vi "Perform Checks.vi"(4 "Owner Path (if applicable)":path, 6 "User VI Owner Status":T1, 8 "error in":errorcluster, 10 "Selected Template VI or CTL name (including file extension)":string, 11 "Destination Folder":path) -> (0 "error out":errorcluster)   [LabVIEW 2021]
doc: "Performs a few sanity checks in order to ensure that everything is ok before attempting to create a new VI based on these inputs. In other words, performs input validation.\n\nSanity checks:\n1. Destination folder exists\n2. Destination folder does not already contain a file with the same name and extension as is about to be created\n3. Selected Template VI or CTL exists\n4. Owner Library or Class exists (if applicable, meaning if the User VI was owned by a library or class)\n\nReturns a meaningful, informative error if any of the sanity checks failed."
uses:
  Owner Status (enum).ctl
panel:
  # "Development\ncontrols/indicators useful for development and testing, but which are not outputs of the VI"
  # "Input\nInputs to the VI"
  # "Output\nOutputs of the VI"
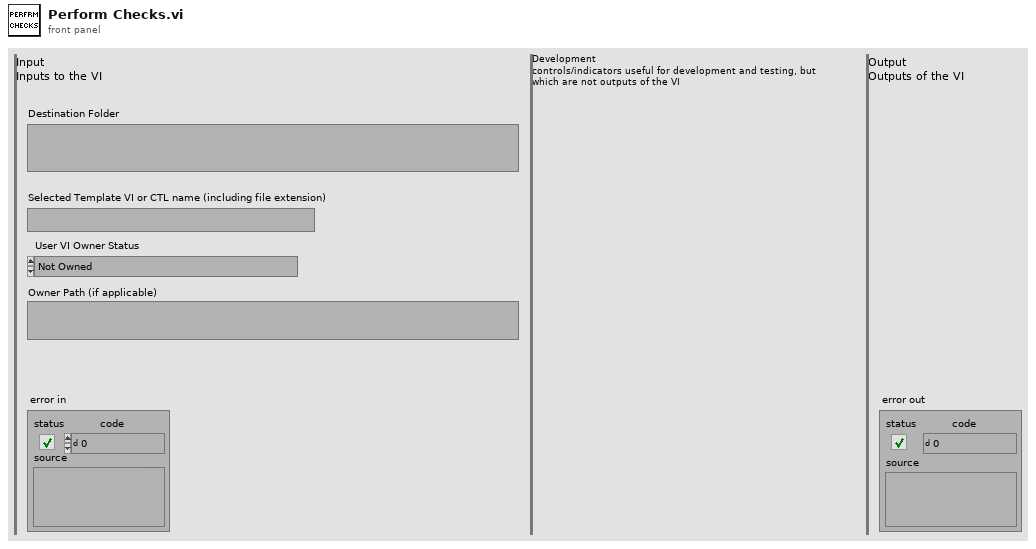
[diagram p1: front panel]
types:
  T1 = typedef "Owner Status (enum).ctl" = enum16{"Not Owned", "Owned by Library (lvlib)", "Owned by Class (lvclass)"}
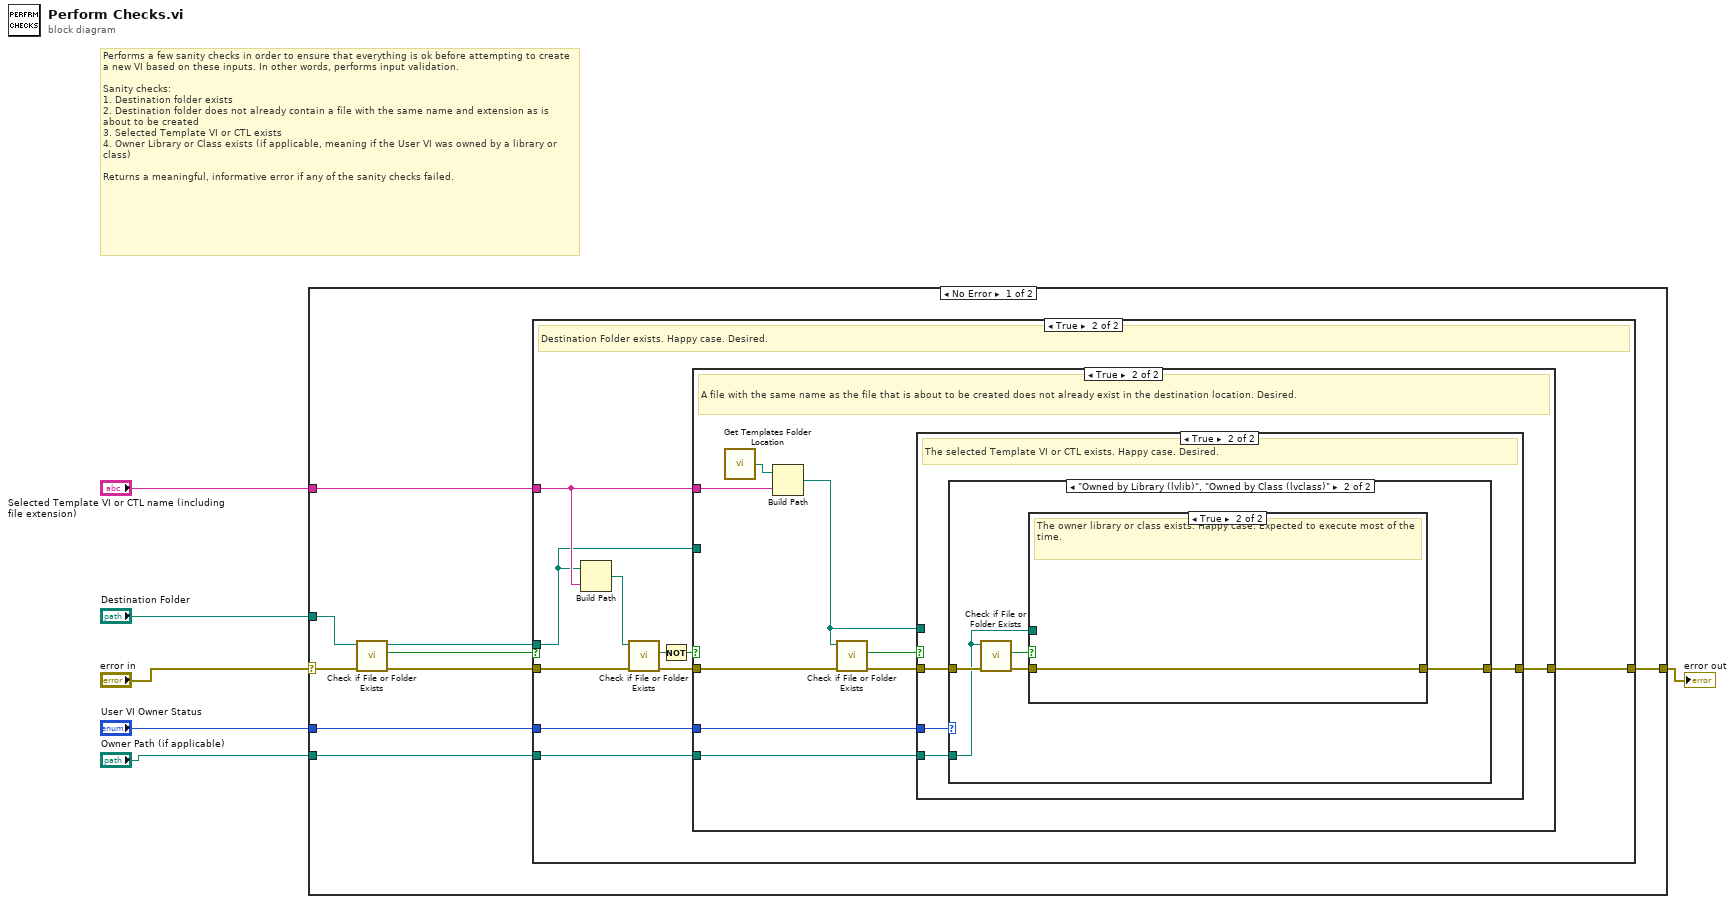
[diagram p0: block diagram]
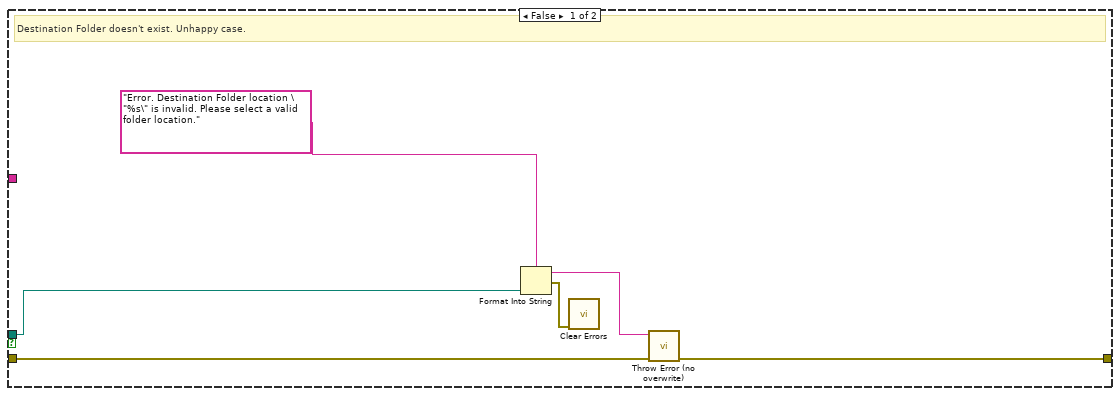
[diagram p2: hidden frame]
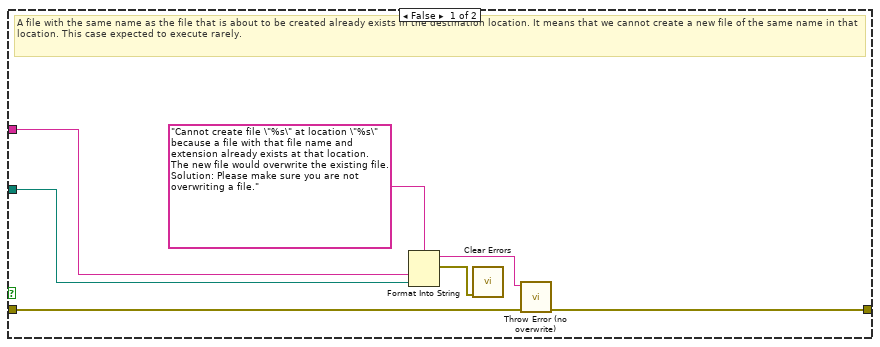
[diagram p3: hidden frame]
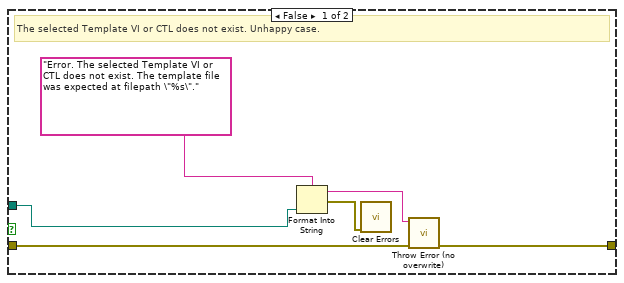
[diagram p4: hidden frame]
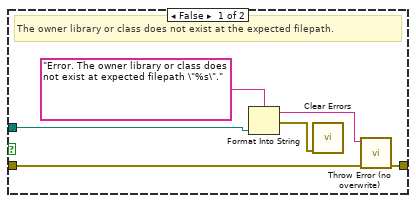
[diagram p6: hidden frame]
diagram:
  # "Performs a few sanity checks in order to ensure that everything is ok before attempting to create a new VI based on these inputs. In other words, performs input validation.\n\nSanity checks:\n1. Destination folder exists\n2. Destination folder does not already contain a file with the same name and extension as is about to be created\n3. Selected Template VI or CTL exists\n4. Owner Library or Class exists (if applicable, meaning if the User VI was owned by a library or class)\n\nReturns a meaningful, informative error if any of the sanity checks failed."
  n1 = case shown="No Error" "error in" {
    selector: "error in" -> [w14 w71]
    tunnel: [w11 w71] -> w5
    tunnel: "Destination Folder" -> [w15 _]
    tunnel: "Selected Template VI or CTL name (including file extension)" -> [w9 _]
    tunnel: "User VI Owner Status" -> [w8 _]
    tunnel: "Owner Path (if applicable)" -> [w7 _]
    frame No Error {
      n2 = call <vilib>:"Check if File or Folder Exists.vi"("error in (no error)"=w14, "path"=w15) -> ("error out"=w13:errorcluster, "file or folder exists?"=w12:bool, "dup path"=w10:path)  [unwired: 7 in]
      n3 = case shown="True" w12 {
        tunnel: w13 -> [w21 w26]
        tunnel: [w20 w31] -> w11
        tunnel: w10 -> [w17 w22]
        tunnel: w9 -> [_ w28]
        tunnel: w8 -> [_ w30]
        tunnel: w7 -> [_ w29]
        frame False {
          # "Destination Folder doesn't exist. Unhappy case."
          n4 = Format Into String(format string="Error. Destination Folder location \"%s\" is invalid. Please select a valid folder location.", w17) -> (resulting string=w16:string, error out=w18:errorcluster)  [unwired: 2 in]
          n5 = call <vilib>:"Clear Errors.vi"("error in (no error)"=w18) -> ()  [unwired: 5 in, 2 out]
          n6 = call "Throw Error (no overwrite).vi"("error in"=w21, "Error Message"=w16) -> ("error out"=w20:errorcluster)  [unwired: 9 in]
        }
        frame True {
          # "Destination Folder exists. Happy case. Desired."
          n7 = Build Path(base path=w22, name or relative path=w28) -> (appended path=w25:path)
          n8 = call <vilib>:"Check if File or Folder Exists.vi"("error in (no error)"=w26, "path"=w25) -> ("error out"=w27:errorcluster, "file or folder exists?"=w24:bool)  [unwired: 7 in, 1 out]
          n9 = Not(x=w24) -> (.not. x?=w23:bool)
          n10 = case shown="True" w23 {
            tunnel: w28 -> [w33 w46]
            tunnel: w27 -> [w35 w45]
            tunnel: [w34 w41] -> w31
            tunnel: w30 -> [_ w40]
            tunnel: w29 -> [_ w39]
            tunnel: w22 -> [w32 _]
            frame False {
              # "A file with the same name as the file that is about to be created already exists in the destination location. It means that we cannot create a new file of the same name in that location. This case expected to execute rarely."
              n11 = Format Into String(format string="Cannot create file \"%s\" at location \"%s\" because a file with that file name and extension already exists at that location. The new file would overwrite the existing file. Solution: Please make sure you are not overwriting a file.", w33, w32) -> (resulting string=w36:string, error out=w37:errorcluster)  [unwired: 2 in]
              n12 = call <vilib>:"Clear Errors.vi"("error in (no error)"=w37) -> ()  [unwired: 5 in, 2 out]
              n13 = call "Throw Error (no overwrite).vi"("error in"=w35, "Error Message"=w36) -> ("error out"=w34:errorcluster)  [unwired: 9 in]
            }
            frame True {
              # "A file with the same name as the file that is about to be created does not already exist in the destination location. Desired."
              n14 = call "Get Templates Folder Location.vi"() -> ("Templates Folder Location"=w47:path)
              n15 = Build Path(base path=w47, name or relative path=w46) -> (appended path=w42:path)
              n16 = call <vilib>:"Check if File or Folder Exists.vi"("error in (no error)"=w45, "path"=w42) -> ("error out"=w44:errorcluster, "file or folder exists?"=w43:bool)  [unwired: 7 in, 1 out]
              n17 = case shown="True" w43 {
                tunnel: w44 -> [w53 w57]
                tunnel: w42 -> [w49 _]
                tunnel: [w48 w56] -> w41
                tunnel: w40 -> [_ w55]
                tunnel: w39 -> [_ w54]
                frame False {
                  # "The selected Template VI or CTL does not exist. Unhappy case."
                  n18 = Format Into String(format string="Error. The selected Template VI or CTL does not exist. The template file was expected at filepath \"%s\".", w49) -> (resulting string=w50:string, error out=w51:errorcluster)  [unwired: 2 in]
                  n19 = call <vilib>:"Clear Errors.vi"("error in (no error)"=w51) -> ()  [unwired: 5 in, 2 out]
                  n20 = call "Throw Error (no overwrite).vi"("error in"=w53, "Error Message"=w50) -> ("error out"=w48:errorcluster)  [unwired: 9 in]
                }
                frame True {
                  # "The selected Template VI or CTL exists. Happy case. Desired."
                  n21 = case shown="\"Owned by Library (lvlib)\", \"Owned by Class (lvclass)\"" w55 {
                    tunnel: w57 -> [w58 w63]
                    tunnel: [w58 w61] -> w56
                    tunnel: w54 -> [_ w59]
                    frame "Not Owned" {
                    }
                    frame "Owned by Library (lvlib)", "Owned by Class (lvclass)" {
                      n22 = call <vilib>:"Check if File or Folder Exists.vi"("error in (no error)"=w63, "path"=w59) -> ("error out"=w62:errorcluster, "file or folder exists?"=w60:bool)  [unwired: 7 in, 1 out]
                      n23 = case shown="True" w60 {
                        tunnel: w62 -> [w66 w70]
                        tunnel: [w65 w70] -> w61
                        tunnel: w59 -> [w64 _]
                        frame False {
                          # "The owner library or class does not exist at the expected filepath."
                          n24 = Format Into String(format string="Error. The owner library or class does not exist at expected filepath \"%s\".", w64) -> (resulting string=w67:string, error out=w68:errorcluster)  [unwired: 2 in]
                          n25 = call <vilib>:"Clear Errors.vi"("error in (no error)"=w68) -> ()  [unwired: 5 in, 2 out]
                          n26 = call "Throw Error (no overwrite).vi"("error in"=w66, "Error Message"=w67) -> ("error out"=w65:errorcluster)  [unwired: 9 in]
                        }
                        frame True {
                          # "The owner library or class exists. Happy case. Expected to execute most of the time."
                        }
                      }
                    }
                  }
                }
              }
            }
          }
        }
      }
    }
    frame Error {
    }
  }
  "error out" <- w5
